vi "Controller LNLS Control PS Communication Loop.vi"(7 "Sync Objects":T1, 8 "error in (no error)":errorcluster, 11 "FOFB Configuration":T5={"FOFB Parameters"={"Network"={"FOFB Controller IP"="", "LNLS Control Network IP"="", "LNLS Control Network Power Supplies TCP Port"=0, "LNLS Control Network FOFB Configuration TCP Port"=0, "Data Server TCP Port"=0, "Monitoring Data TCP Port"=0, "Configuration GUI TCP Port"=0, "TCP Listening Timeout"=0}, "Fast Acquisition"={"Acquisition Period"=0, "Data Buffer Size"=0}, "Response Matrix Measurement"={"Step Amplitude"=0.0, "Time Between Steps"=0, "Step Duration"=0, "Number of Averages"=0}, "Correction Algorithm"={"Correction Period"=0, "Reference Orbit Path"=path "", "Response Matrix Path"=path "", "Correction Matrix Path"=path "", "Horizontal Correction Factor"=0.0, "Vertical Correction Factor"=0.0, "Beam Current FOFB Threshold"=0.0, "Decouple H-V"=FALSE}, "Acquisition Network"=[], "Actuation Network"=[]}, "Number of Acquisition Chassis"=0, "Number of Actuation Chassis"=0, "Number of BPM Readings"=0, "BPM Reading Names"=[], "Selected BPM Readings"=[0, 1, 2, 3, 4, 5, 6, 7, 8, 9, 10, 11, 12, 13, 14, 15, 16, 17, 18, 19, 20, 21, 22, 23, 24, 25, 26, 27, 28, 29, 30, 31, 32, 33, 34, 35, 36, 37, 38, 39, 40, 41, 42, 43, 44, 45, 46, 47, 48, 49], "Number of Correctors"=0, "Corrector Names"=[], "Selected Correctors"=[0, 1, 2, 3, 4, 5, 6, 7, 8, 9, 10, 11, 12, 13, 14, 15, 16, 17, 18, 19, 20, 21, 22, 23, 24, 25, 26, 27, 28, 29, 30, 31, 32, 33, 34, 35, 36, 37, 38, 39, 40, 41, 42, 43, 44, 45, 46, 47, 48, 49], "Reference Orbit"=[], "Response Matrix"=[], "Correction Matrix"=[], "Acquisition Chassis Names"=[], "Actuation Chassis Names"=[], "Acquisition Variables"=[], "Actuation Variables"=[], "PS Matrix Mapping"=[], "Inverse PS Matrix Mapping"=[], "Response Matrix Beam Energy (MeV)"=0.0, "PID Parameters"=[], "BPM Planes"=[], "Corrector Planes"=[], "RMM Step Factor"=[]}) -> (0 "error out":errorcluster)   [LabVIEW 2011, in "Controller VIs.lvlib"]
uses:
  Controller VIs.lvlib
  Types Definitions/Type FOFB Configuration.ctl
  Types Definitions/Type FOFB Parameters.ctl
  Types Definitions/Type Network Configuration.ctl
  Types Definitions/Type FA Configuration.ctl
  Types Definitions/Type Response Matrix Measurement Configuration.ctl
  Types Definitions/Type Correction Algorithm Configuration.ctl
  Types Definitions/Type Acquisition Network Configuration.ctl
  Types Definitions/Type Actuation Network Configuration.ctl
  Types Definitions/Type PID Parameters.ctl
  Types Definitions/Type Synchronization Objects.ctl
  Types Definitions/Type Blocking Synchronization Objects.ctl
  Types Definitions/Type FA Request Parameters.ctl
  Types Definitions/Type BPM and PS select cluster.ctl
  Types Definitions/Type FA File Parameters.ctl
  Types Definitions/Type Monitoring Data.ctl
  Types Definitions/Type Diagnostics Data.ctl
  Types Definitions/Type CPU Loads Array.ctl
  Types Definitions/Type CPU Loads.ctl
  Types Definitions/Type Non-blocking Synchronization Objects.ctl
  Types Definitions/Type FOFB Variables.ctl
  Types Definitions/Type Actuation State.ctl
  <vilib>/Platform/TimedLoop/XDataNode/timing_clust.ctl
  <vilib>/Platform/TimedLoop/XDataNode/nitl_modes.ctl
  <vilib>/Platform/TimedLoop/XDataNode/wakeup.ctl
  Controller Global Variables/Monitoring Data.vi
  <vilib>/Platform/TimedLoop/XDataNode/XDataNode.xnode
  LNLS Control VIs.lvlib
  Common VIs.lvlib
  Misc VIs.lvlib
  Controller Global Variables.lvlib
  <vilib>/Platform/TimedLoop/XDataNode/XDNodeRunTimeDep.lvlib
  Log VIs.lvlib
  Type Definitions.lvlib
panel:
  out "Comando 1":u8[](array[numeric])
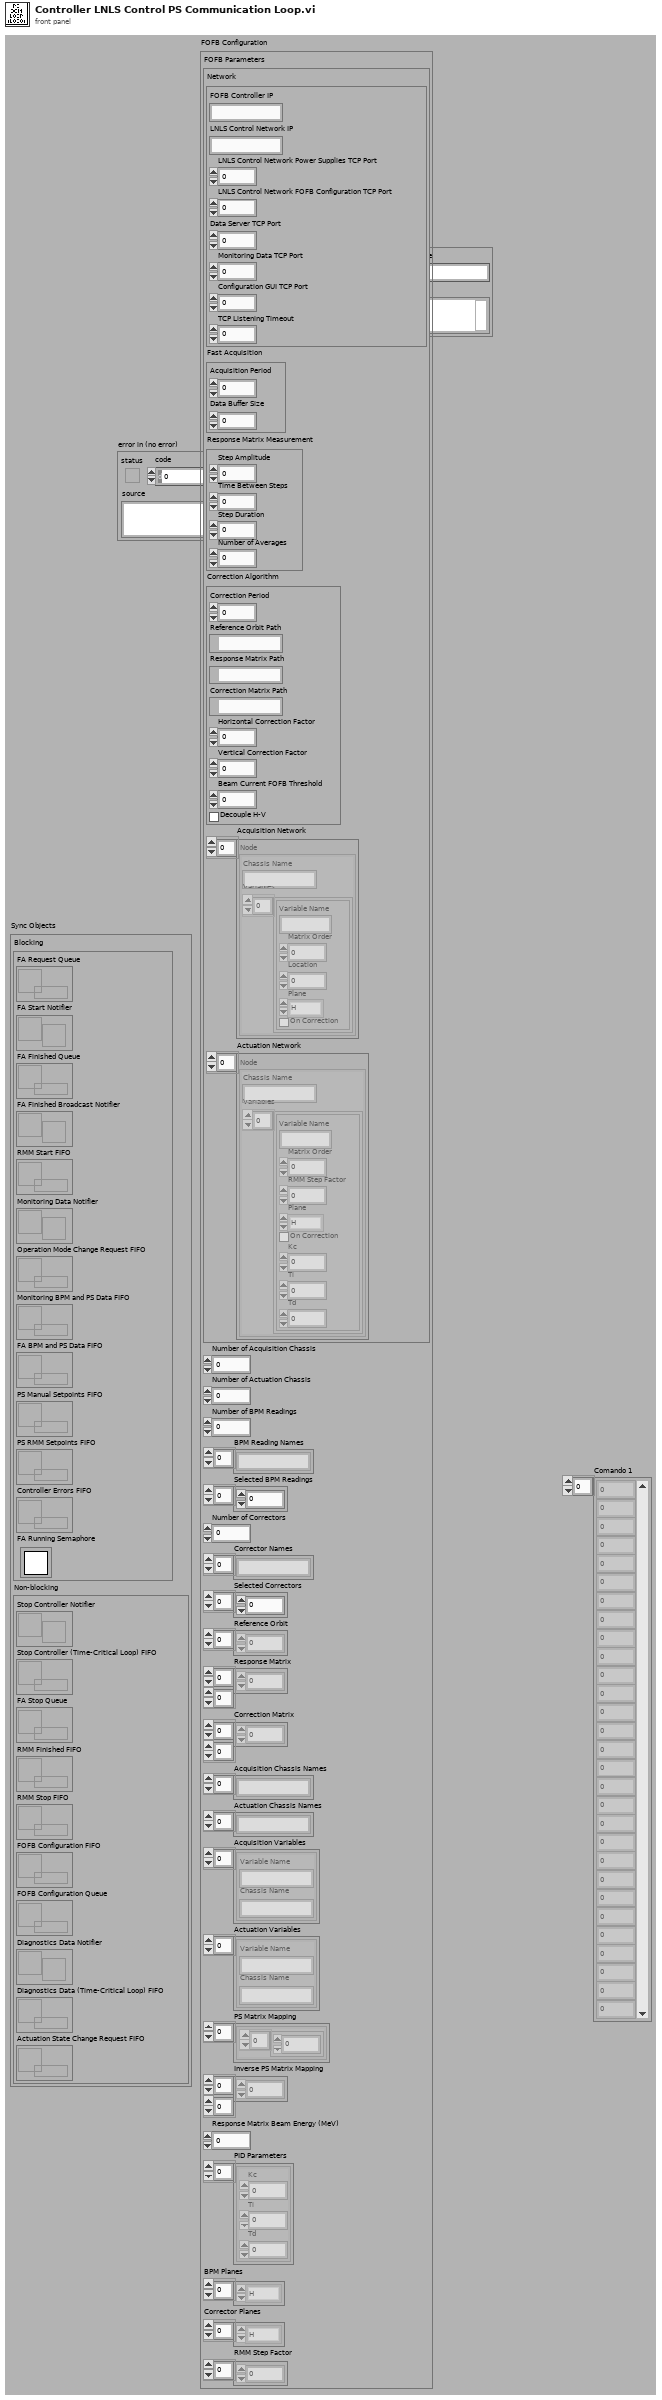
[diagram p1: front panel]
types:
  T1 = typedef "Type Definitions.lvlib/Type Synchronization Objects.ctl" = cluster{"Blocking":T2, "Non-blocking":T4}
  T2 = typedef "Type Definitions.lvlib/Type Blocking Synchronization Objects.ctl" = cluster{"FA Request Queue":refnum<queue>, "FA Start Notifier":refnum<notifier>, "FA Finished Queue":refnum<queue>, "FA Finished Broadcast Notifier":refnum<notifier>, "RMM Start FIFO":refnum<k33>, "Monitoring Data Notifier":refnum<notifier>, "Operation Mode Change Request FIFO":refnum<k33>, "Monitoring BPM and PS Data FIFO":refnum<k33>, "FA BPM and PS Data FIFO":refnum<k33>, "PS Manual Setpoints FIFO":refnum<k33>, "PS RMM Setpoints FIFO":refnum<k33>, "Controller Errors FIFO":refnum<k33>, "FA Running Semaphore":T3}
  T3 = typedef "Semaphore RefNum" = refnum<k1>
  T4 = typedef "Type Definitions.lvlib/Type Non-blocking Synchronization Objects.ctl" = cluster{"Stop Controller Notifier":refnum<notifier>, "Stop Controller (Time-Critical Loop) FIFO":refnum<k33>, "FA Stop Queue":refnum<queue>, "RMM Finished FIFO":refnum<k33>, "RMM Stop FIFO":refnum<k33>, "FOFB Configuration FIFO":refnum<k33>, "FOFB Configuration Queue":refnum<queue>, "Diagnostics Data Notifier":refnum<notifier>, "Diagnostics Data (Time-Critical Loop) FIFO":refnum<k33>, "Actuation State Change Request FIFO":refnum<k33>}
  T5 = typedef "Type Definitions.lvlib/Type FOFB Configuration.ctl" = cluster{"FOFB Parameters":T6, "Number of Acquisition Chassis":i32, "Number of Actuation Chassis":i32, "Number of BPM Readings":i32, "BPM Reading Names":string[], "Selected BPM Readings":u32[], "Number of Correctors":i32, "Corrector Names":string[], "Selected Correctors":u32[], "Reference Orbit":dbl[], "Response Matrix":dbl[][], "Correction Matrix":dbl[][], "Acquisition Chassis Names":string[], "Actuation Chassis Names":string[], "Acquisition Variables":cluster{"Variable Name":string, "Chassis Name":string}[], "Actuation Variables":cluster{"Variable Name":string, "Chassis Name":string}[], "PS Matrix Mapping":cluster{u32[]}[], "Inverse PS Matrix Mapping":u32[][], "Response Matrix Beam Energy (MeV)":dbl, "PID Parameters":T13[], "BPM Planes":enum8{"H", "V"}[], "Corrector Planes":enum8{"H", "V"}[], "RMM Step Factor":dbl[]}
  T6 = typedef "Type Definitions.lvlib/Type FOFB Parameters.ctl" = cluster{"Network":T7, "Fast Acquisition":T8, "Response Matrix Measurement":T9, "Correction Algorithm":T10, "Acquisition Network":T11, "Actuation Network":T12}
  T7 = typedef "Type Definitions.lvlib/Type Network Configuration.ctl" = cluster{"FOFB Controller IP":string, "LNLS Control Network IP":string, "LNLS Control Network Power Supplies TCP Port":u16, "LNLS Control Network FOFB Configuration TCP Port":u16, "Data Server TCP Port":u16, "Monitoring Data TCP Port":u16, "Configuration GUI TCP Port":u16, "TCP Listening Timeout":i32}
  T8 = typedef "Type Definitions.lvlib/Type FA Configuration.ctl" = cluster{"Acquisition Period":u32, "Data Buffer Size":u32}
  T9 = typedef "Type Definitions.lvlib/Type Response Matrix Measurement Configuration.ctl" = cluster{"Step Amplitude":dbl, "Time Between Steps":u32, "Step Duration":u32, "Number of Averages":u32}
  T10 = typedef "Type Definitions.lvlib/Type Correction Algorithm Configuration.ctl" = cluster{"Correction Period":u32, "Reference Orbit Path":path, "Response Matrix Path":path, "Correction Matrix Path":path, "Horizontal Correction Factor":dbl, "Vertical Correction Factor":dbl, "Beam Current FOFB Threshold":dbl, "Decouple H-V":bool}
  T11 = typedef "Type Definitions.lvlib/Type Acquisition Network Configuration.ctl" = cluster{"Chassis Name":string, "Variables":cluster{"Variable Name":string, "Matrix Order":u32, "Location":dbl, "Plane":enum8{"H", "V"}, "On Correction":bool}[]}[]
  T12 = typedef "Type Definitions.lvlib/Type Actuation Network Configuration.ctl" = cluster{"Chassis Name":string, "Variables":cluster{"Variable Name":string, "Matrix Order":u32, "RMM Step Factor":dbl, "Plane":enum8{"H", "V"}, "On Correction":bool, "Kc":dbl, "Ti":dbl, "Td":dbl}[]}[]
  T13 = typedef "Type Definitions.lvlib/Type PID Parameters.ctl" = cluster{"Kc":fxp<+/-,16,8>, "Ti":fxp<+/-,16,8>, "Td":fxp<+/-,16,8>}
  T14 = enum16{"Wait Connection", "Read Data", "Write Data", "Close Connection", "Idle"}
  T15 = typedef "XDNodeRunTimeDep.lvlib/timing_clust.ctl" = cluster{"Expected End [f-1]":u64, "Actual End [f-1]":u64, "Finished Late? [f-1]":bool, "Expected End [i-1]":u64, "Actual End [i-1]":u64, "Finished Late? [i-1]":bool, "Expected Start [i]":u64, "Actual Start [i]":u64, "Expected Start [f]":u64, "Actual Start [f]":u64, "Source Name":string, "Structure Name":string, "Period":i64, "Deadline":i64, "Offset":i64, "Start":i64, "Priority":i32, "Timeout":i32, "Mode":T16, "Wakeup Reason":T17, "Error":errorcluster, "Source Type":string, "Secondary Source Type":string, "Global End Time":u64, "Global Start Time":u64, "Frame Duration":u64, "Iteration Duration":u64, "Assigned CPU":i32, "I/O Scan Engine Mode":u32}
  T16 = typedef "XDNodeRunTimeDep.lvlib/nitl_modes.ctl" = enum32{"No Change", "Process missed periods, maintain original phase", "Discard missed periods, maintain original phase", "Process missed periods, ignore original phase", "Discard missed periods, ignore original phase"}
  T17 = typedef "XDNodeRunTimeDep.lvlib/wakeup.ctl" = enum32{"Normal", "Aborted", "Asynchronous wakeup", "Timing source error", "Timed loop error", "Timeout"}
  T18 = enum16{"open", "replace", "create", "open or create", "replace or create", "replace or create with confirmation"}
  T19 = typedef "Type Definitions.lvlib/Type Monitoring Data.ctl" = cluster{"Timestamp":timestamp, "BPM Readings":dbl[], "PS Readings":dbl[], "PS FOFB Setpoints":dbl[], "PS Status per Rack":u8[], "PS ON-OFF per Rack":u8[], "Operation Mode":enum16{"Idle Mode", "Error Mode", "Manual Mode", "FOFB Mode", "RMM Mode"}, "Diagnostics Data":T20, "Controller Status Table":i32[]}
  T20 = typedef "Type Definitions.lvlib/Type Diagnostics Data.ctl" = cluster{"Time-Critical Loop Missed Iterations":u32, "Time-Critical Loop Execution Time (usec)":u32, "FA Buffer Usage":u32, "Available Memory (bytes)":u32, "CPU Loads Array":T21}
  T21 = typedef "Type Definitions.lvlib/Type CPU Loads Array.ctl" = T22[]
  T22 = typedef "Type Definitions.lvlib/Type CPU Loads.ctl" = cluster{"Total (%)":dbl, "Time Critical (%)":dbl, "Timed Structures (%)":dbl, "High (%)":dbl, "Above Normal (%)":dbl, "Normal (%)":dbl, "Background (%)":dbl, "Idle (%)":dbl, "ISR (%)":dbl}
  T23 = typedef "Type Definitions.lvlib/Type LOCON_BIPOLAR_16BITS.ctl" = cluster{"priority":u8, "flag":u8, "analog value":u16, "status":u8}
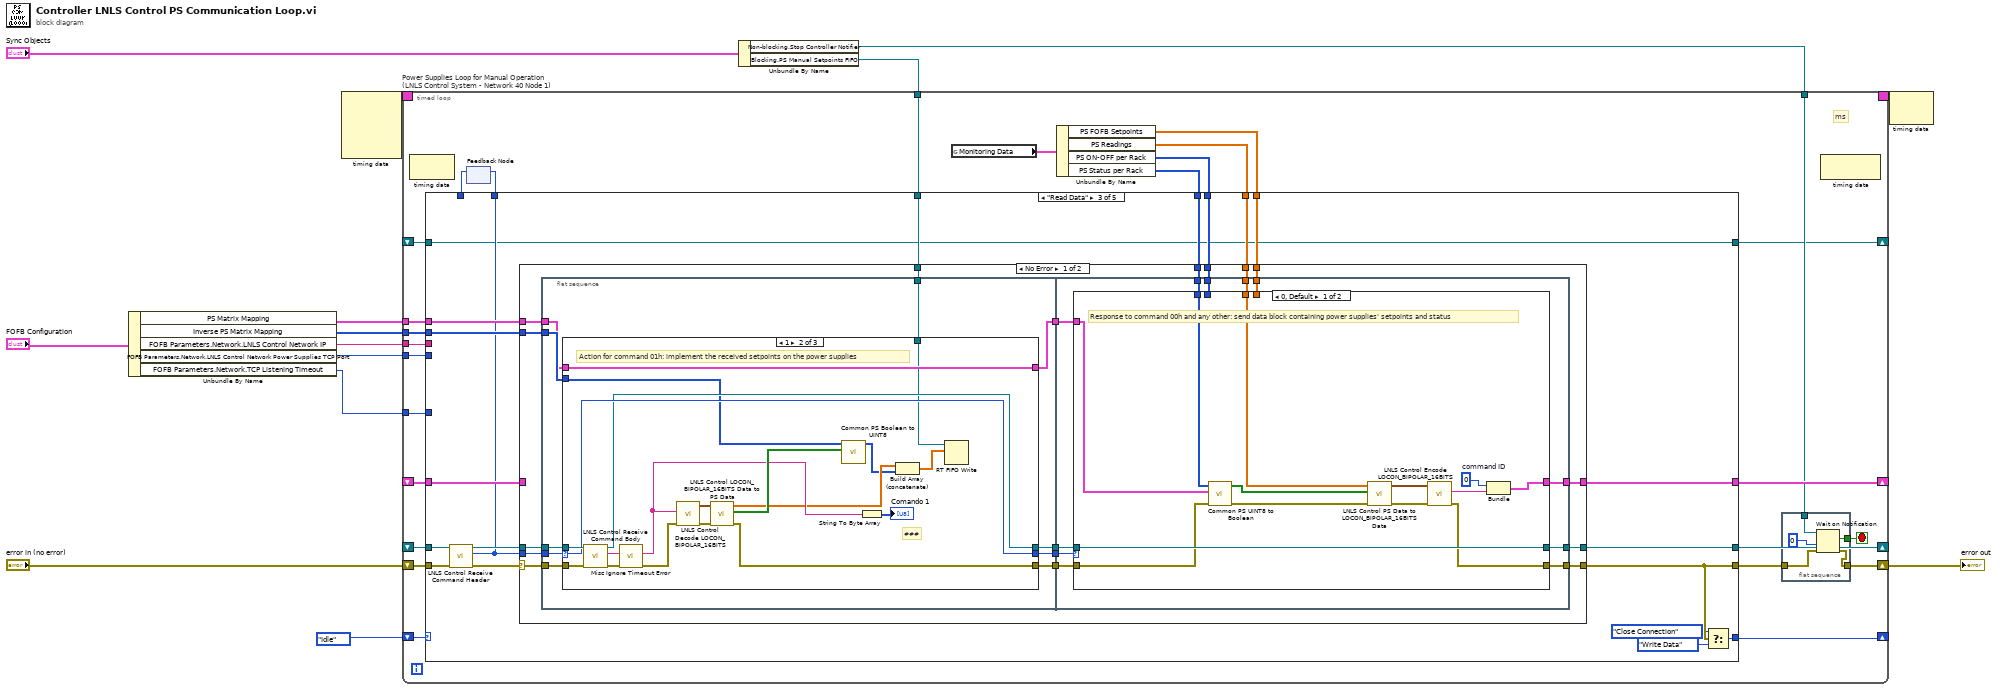
[diagram p0: block diagram]
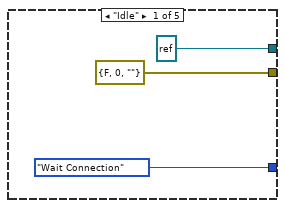
[diagram p2: hidden frame]
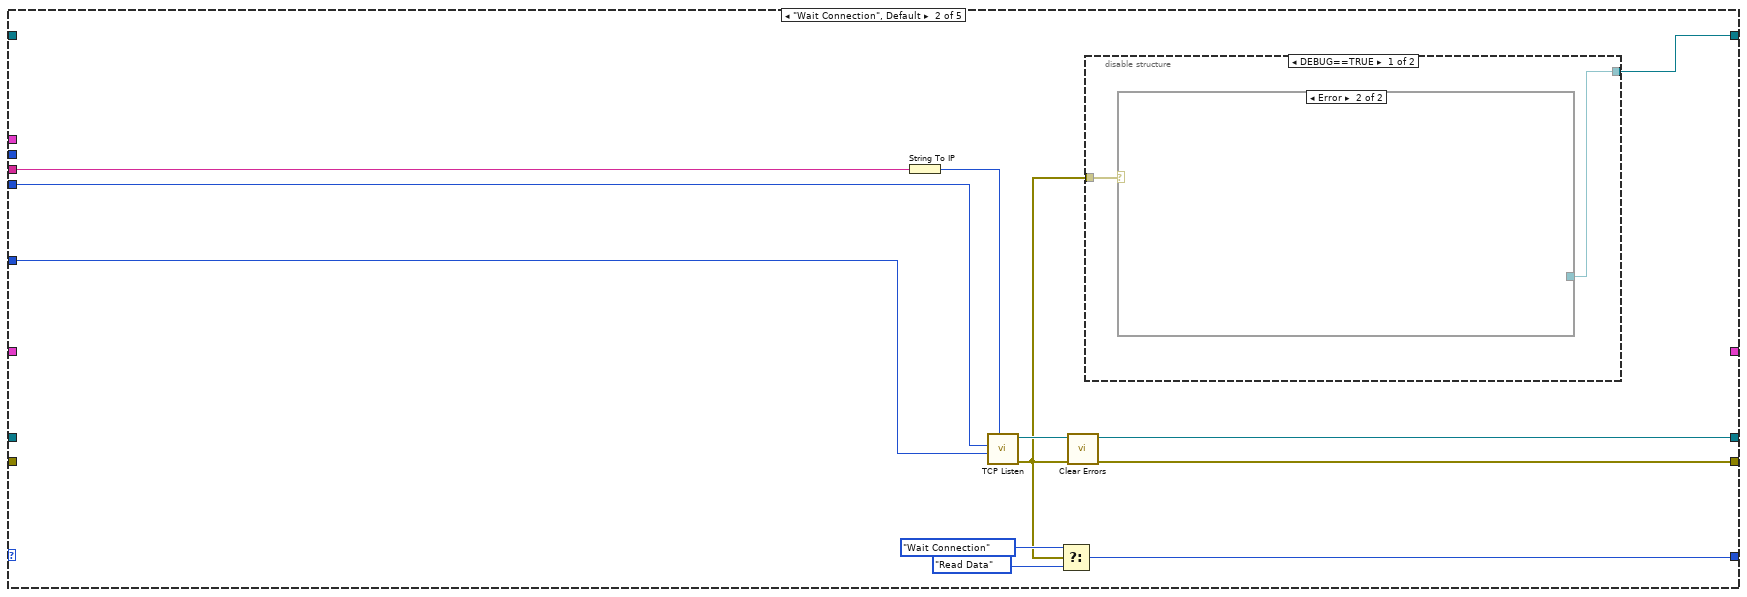
[diagram p3: hidden frame]
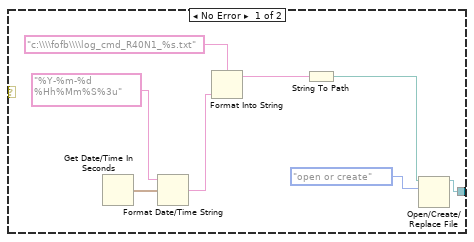
[diagram p4: hidden frame]
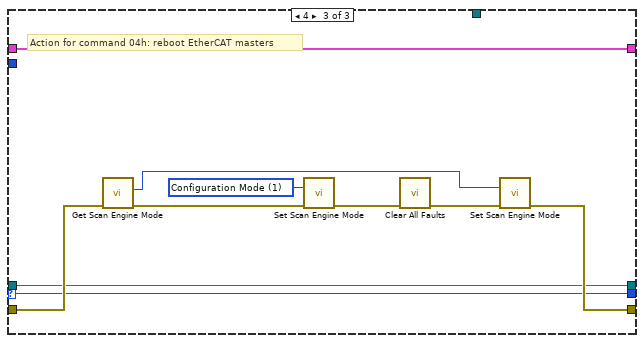
[diagram p7: hidden frame]
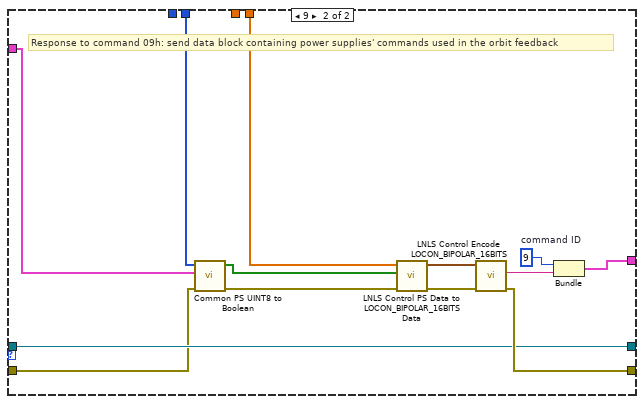
[diagram p8: hidden frame]
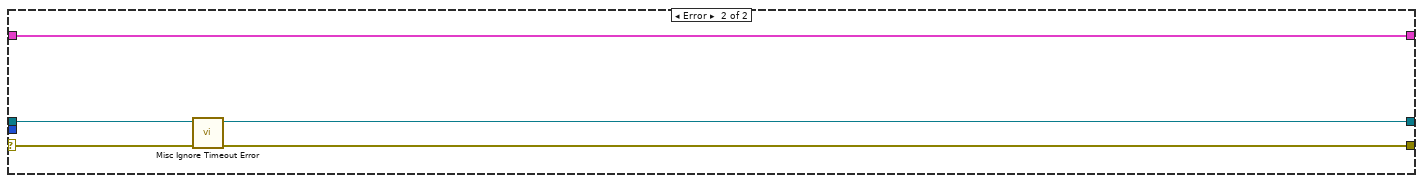
[diagram p9: hidden frame]
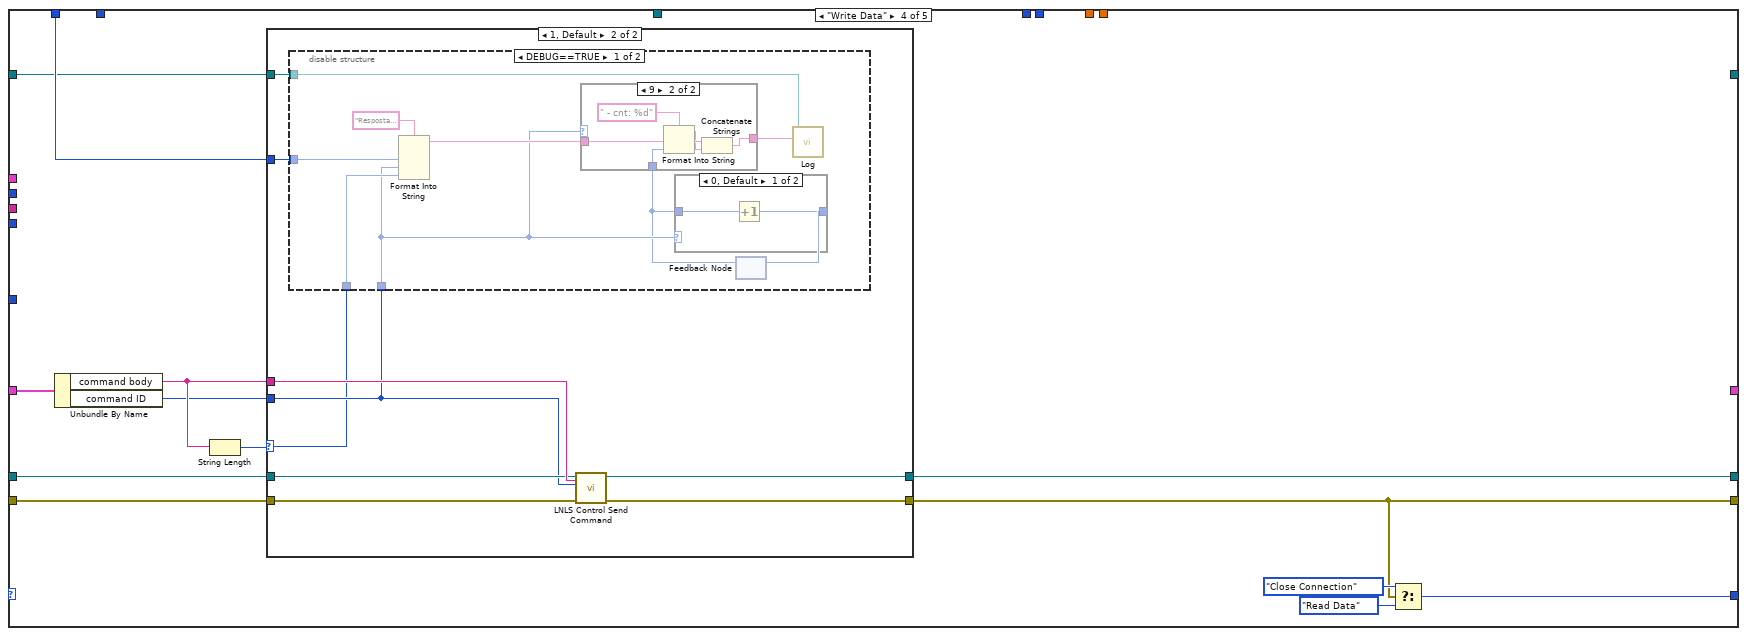
[diagram p10: hidden frame]
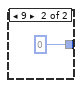
[diagram p13: hidden frame]
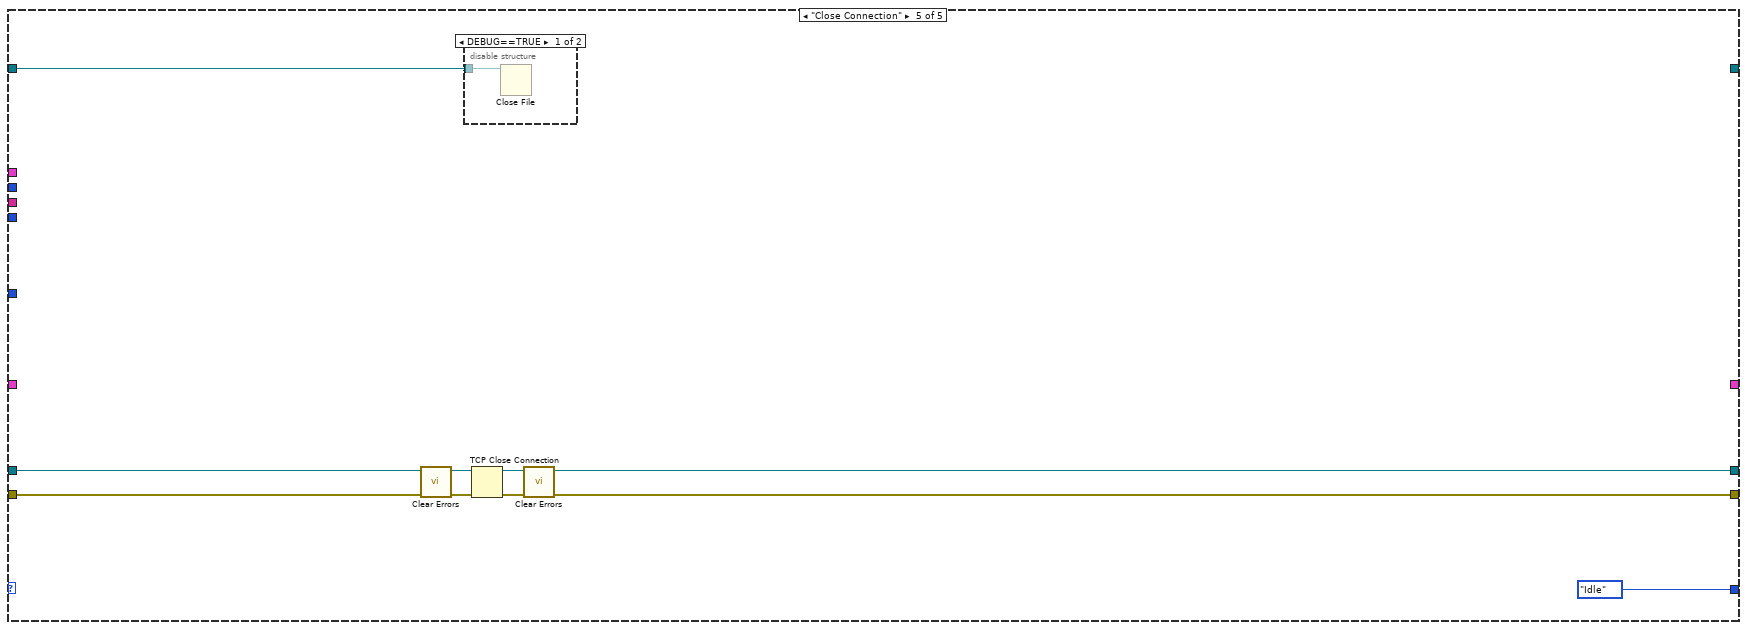
[diagram p15: hidden frame]
diagram:
  n1 = Unbundle By Name("FOFB Configuration") -> ("PS Matrix Mapping"=w7:cluster{u32[]}[], "Inverse PS Matrix Mapping"=w8:u32[][], "FOFB Parameters.Network.LNLS Control Network IP"=w9:string, "FOFB Parameters.Network.LNLS Control Network Power Supplies TCP Port"=w6:u16, "FOFB Parameters.Network.TCP Listening Timeout"=w4:i32)
  n2 = node-c288() -> (w2:T15)  [unwired: 4 in]
  n3 = Unbundle By Name("Sync Objects") -> ("Non-blocking.Stop Controller Notifier"=w5:refnum<notifier>, "Blocking.PS Manual Setpoints FIFO"=w3:refnum<k33>)
  n4 = timed-loop "Power Supplies Loop for Manual Operation (LNLS Control System - Network 40 Node 1)" {
    shift-right: [w38] -> _
    shift-left: T14."Idle" ("f") -> [w40]
    shift-right: [w39] -> _
    shift-left: _ -> [w37]
    shift-right: [w25] -> w12
    shift-left: "error in (no error)" -> [w33]
    shift-right: [w35] -> _
    shift-left: _ -> [w34]
    tunnel: w6 -> [w36]
    tunnel: w9 -> [w32]
    tunnel: w8 -> [w31]
    tunnel: w7 -> [w30]
    tunnel: w5 -> [w28]
    tunnel: w4 -> [w29]
    tunnel: w3 -> [w21]
    timing: w2 -> [_]
    timing-out: [_] -> w1
    shift-right: [w16] -> _
    shift-left: _ -> [w15]
    stop <- w27 stop-if-true
    # "ms"
    n5 = node-c288() -> ()  [unwired: 1 in, 1 out]
    n6 = feedback #1() -> (w17:u8)  [unwired: 1 in]
    n7 = global read "Monitoring Data.vi" "Monitoring Data"() -> (w22:T19)
    n8 = Unbundle By Name(w22) -> ("PS FOFB Setpoints"=w24:dbl[], "PS Readings"=w23:dbl[], "PS ON-OFF per Rack"=w19:u8[], "PS Status per Rack"=w20:u8[])
    n9 = case shown="\"Read Data\"" w40 {
      tunnel: [refnum<k5> refnum ("connection ID") w57 w91 w197 w240] -> w39
      tunnel: [errorcluster {"status"=FALSE, "code"=0, "source"=""} ("error out") w60 w89 w196 w237] -> w26
      tunnel: [T14."Wait Connection" w61 w90 w202 T14."Idle"] -> w38
      tunnel: w37 -> [_ _ w87 w199 w241]
      tunnel: w33 -> [_ _ w88 w198 w235]
      tunnel: w36 -> [_ w56 _ _ _]
      tunnel: [_ _ w84 _ _] -> w35
      tunnel: w34 -> [_ _ w82 w201 _]
      tunnel: w32 -> [_ w54 _ _ _]
      tunnel: w31 -> [_ _ w80 _ _]
      tunnel: w30 -> [_ _ w79 _ _]
      tunnel: w29 -> [_ w53 _ _ _]
      tunnel: w24 -> [_ _ w78 _ _]
      tunnel: w23 -> [_ _ w77 _ _]
      tunnel: w20 -> [_ _ w76 _ _]
      tunnel: w21 -> [_ _ w75 _ _]
      tunnel: w19 -> [_ _ w74 _ _]
      tunnel: w17 -> [_ _ _ w194 _]
      tunnel: [_ _ w73 _ _] -> w18
      tunnel: [_ w52 w72 _ _] -> w16
      tunnel: w15 -> [_ _ w72 w193 w234]
      frame "Idle" {
      }
      frame "Wait Connection", Default {
        n10 = String To IP(1:w54) -> (0:w55:u32)
        n11 = call <vilib>:"TCP Listen.vi"("net address"=w55, "timeout ms (wait forever: -1)"=w53, "port"=w56) -> ("error out"=w51:errorcluster, "connection ID"=w57:refnum<k5>)  [unwired: 4 in, 3 out]
        n12 = Select(t=T14."Wait Connection", s=w51, f=T14."Read Data") -> (s? t:f=w61:T14)
        n13 = call <vilib>:"Clear Errors.vi"("error in (no error)"=w51) -> ("error out"=w60:errorcluster)  [unwired: 6 out]
        n14 = disable-structure shown="DEBUG==TRUE" {
          disable-tunnel: [w63 _] -> w52
          disable-tunnel: w51 -> [w62 _]
          frame condition #0 {
            n15 = case shown="Error" w62 {
              tunnel: [w64 _] -> w63
              frame No Error {
                n16 = Get Date/Time In Seconds() -> (seconds since 1Jan1904=w67:timestamp)
                n17 = Format Date/Time String(time format string (%c)="%Y-%m-%d %Hh%Mm%S%3u", seconds (now)=w67) -> (date/time string=w65:string)  [unwired: 1 in]
                n18 = Format Into String(format string="c:\\\\fofb\\\\log_cmd_R40N1_%s.txt", w65) -> (resulting string=w69:string)  [unwired: 2 in, 1 out]
                n19 = String To Path(string=w69) -> (path=w68:path)
                n20 = Open/Create/Replace File(file path (use dialog)=w68, operation (0:open)=T18."open or create") -> (refnum out=w64:refnum<file>)  [unwired: 4 in, 2 out]
              }
              frame Error {
              }
            }
          }
          frame condition #1 (active) {
          }
        }
      }
      frame "Read Data" {
        n21 = call "LNLS Control Receive Command Header.vi"("error in (no error)"=w88, "connection ID"=w87) -> ("error out"=w83:errorcluster, "command ID"=w73:u8, "connection ID out"=w86:refnum<k5>)  [unwired: 7 in]
        n22 = case shown="No Error" w83 {
          selector: w83 -> [w103 w188]
          tunnel: [w108 w191] -> w91
          tunnel: [w107 w189] -> w89
          tunnel: w86 -> [w106 w191]
          tunnel: w73 -> [w105 _]
          tunnel: [w104 w190] -> w84
          tunnel: w82 -> [_ w190]
          tunnel: w80 -> [w99 _]
          tunnel: w79 -> [w97 _]
          tunnel: w78 -> [w96 _]
          tunnel: w77 -> [w95 _]
          tunnel: w76 -> [w94 _]
          tunnel: w75 -> [w93 _]
          tunnel: w74 -> [w92 _]
          frame No Error {
            n23 = flat-sequence {
              tunnel: [w118] -> w102
              tunnel: [w117] -> w101
              tunnel: w106 -> [w116]
              tunnel: w105 -> [w115]
              tunnel: w103 -> [w114]
              tunnel: [w113] -> w100
              tunnel: w99 -> [w112]
              tunnel: [w111] -> w98
              tunnel: w97 -> [w110]
              tunnel: w93 -> [w109]
              tunnel: [w158] -> w108
              tunnel: w102 -> [w157]
              tunnel: [w161] -> w107
              tunnel: w101 -> [w160]
              tunnel: [w156] -> w104
              tunnel: w100 -> [w159]
              tunnel: w98 -> [w155]
              tunnel: w96 -> [w154]
              tunnel: w95 -> [w153]
              tunnel: w94 -> [w152]
              tunnel: w92 -> [w151]
              frame #0 {
                n24 = case shown="1" w115 {
                  selector: w115 -> [w120 w137 w143]
                  tunnel: w114 -> [w122 w139 w150]
                  tunnel: [w122 w138 w149] -> w117
                  tunnel: [w121 w136 w142] -> w118
                  tunnel: w116 -> [w121 w140 w142]
                  tunnel: [w120 w137 w143] -> w113
                  tunnel: w112 -> [_ w135 _]
                  tunnel: [w119 w134 w141] -> w111
                  tunnel: w110 -> [w119 w134 w141]
                  tunnel: w109 -> [_ w126 _]
                  frame 0, Default {
                  }
                  frame 1 {
                    # "###"
                    # "Action for command 01h: implement the received setpoints on the power supplies"
                    n25 = call "LNLS Control Receive Command Body.vi"("error in (no error)"=w139, "connection ID"=w140) -> ("error out"=w130:errorcluster, "command body"=w128:string, "connection ID out"=w136:refnum<k5>)  [unwired: 6 in, 1 out]
                    n26 = call "Misc Ignore Timeout Error.vi"("error in (no error)"=w130) -> ("error out"=w129:errorcluster)  [unwired: 10 in]
                    n27 = call "LNLS Control Decode LOCON_BIPOLAR_16BITS.vi"("error in (no error)"=w129, "command body"=w128) -> ("error out"=w133:errorcluster, "LOCON data"=w132:T23[])  [unwired: 6 in]
                    n28 = call "LNLS Control LOCON_BIPOLAR_16BITS Data to PS Data.vi"("error in (no error)"=w133, "PS Setpoints LOCON Data"=w132) -> ("error out"=w138:errorcluster, "PS Status"=w131:bool[], "PS Setpoints"=w125:dbl[])  [unwired: 7 in]
                    n29 = call "Common PS Boolean to UINT8.vi"("PS ON-OFF"=w131, "Inverse PS Matrix Mapping"=w135) -> ("PS ON-OFF (per PS Rack)"=w124:u8[])  [unwired: 8 in, 1 out]
                    n30 = String To Byte Array(string=w128) -> (unsigned byte array=→"Comando 1":u8[])
                    n31 = Build Array (concatenate)(w125, w124) -> (w123:dbl[])
                    n32 = RT FIFO Write(0:w126, 1:w123) -> ()  [unwired: 3 in, 4 out]
                  }
                  frame 4 {
                    w148 = 1 items=["Configuration Mode"=1, "Active Mode"=2] ("mode (Active Mode)")
                    # "Action for command 04h: reboot EtherCAT masters"
                    n33 = call <vilib>:"Get Scan Engine Mode.vi"("error in (no error)"=w150) -> ("error out"=w147:errorcluster, "mode"=w144:i32)  [unwired: 9 in]
                    n34 = call <vilib>:"Set Scan Engine Mode.vi"("mode (Active Mode)"=w148, "error in (no error)"=w147) -> ("error out"=w146:errorcluster)  [unwired: 13 in]
                    n35 = call <vilib>:"Clear All Faults.vi"("error in (no error)"=w146) -> ("error out"=w145:errorcluster)  [unwired: 1 in, 9 out]
                    n36 = call <vilib>:"Set Scan Engine Mode.vi"("mode (Active Mode)"=w144, "error in (no error)"=w145) -> ("error out"=w149:errorcluster)  [unwired: 13 in]
                  }
                }
              }
              frame #1 {
                n37 = case shown="0, Default" w159 {
                  tunnel: w160 -> [w168 w182]
                  tunnel: [w169 w185] -> w161
                  tunnel: [w174 w184] -> w158
                  tunnel: w157 -> [w174 w184]
                  tunnel: [w170 w183] -> w156
                  tunnel: w155 -> [w166 w180]
                  tunnel: w154 -> [_ w178]
                  tunnel: w153 -> [w163 _]
                  tunnel: w152 -> [w162 _]
                  tunnel: w151 -> [_ w175]
                  frame 0, Default {
                    w171 = u8 0  # command ID
                    # "Response to command 00h and any other: send data block containing power supplies' setpoints and status"
                    n38 = call "Common PS UINT8 to Boolean.vi"("error in (no error)"=w168, "PS Matrix Mapping"=w166, "PS Status (per PS Rack)"=w162) -> ("error out"=w165:errorcluster, "PS Status"=w167:bool[])  [unwired: 7 in]
                    n39 = call "LNLS Control PS Data to LOCON_BIPOLAR_16BITS Data.vi"("error in (no error)"=w165, "PS Status"=w167, "PS Readings/Setpoints"=w163) -> ("error out"=w172:errorcluster, "PS Readings/Setpoints LOCON Data"=w173:T23[])  [unwired: 7 in]
                    n40 = call "LNLS Control Encode LOCON_BIPOLAR_16BITS.vi"("error in (no error)"=w172, "LOCON Data"=w173) -> ("error out"=w169:errorcluster, "command body"=w164:string)  [unwired: 8 in]
                    n41 = Bundle("command ID"=w171, "command body"=w164) -> (w170:cluster{"command ID":u8, "command body":string})  [unwired: 1 in]
                  }
                  frame 9 {
                    w186 = u8 9  # command ID
                    # "Response to command 09h: send data block containing power supplies' commands used in the orbit feedback"
                    n42 = call "Common PS UINT8 to Boolean.vi"("error in (no error)"=w182, "PS Matrix Mapping"=w180, "PS Status (per PS Rack)"=w175) -> ("error out"=w179:errorcluster, "PS Status"=w181:bool[])  [unwired: 7 in]
                    n43 = call "LNLS Control PS Data to LOCON_BIPOLAR_16BITS Data.vi"("error in (no error)"=w179, "PS Status"=w181, "PS Readings/Setpoints"=w178) -> ("error out"=w176:errorcluster, "PS Readings/Setpoints LOCON Data"=w177:T23[])  [unwired: 7 in]
                    n44 = call "LNLS Control Encode LOCON_BIPOLAR_16BITS.vi"("error in (no error)"=w176, "LOCON Data"=w177) -> ("error out"=w185:errorcluster, "command body"=w187:string)  [unwired: 8 in]
                    n45 = Bundle("command ID"=w186, "command body"=w187) -> (w183:cluster{"command ID":u8, "command body":string})  [unwired: 1 in]
                  }
                }
              }
            }
          }
          frame Error {
            n46 = call "Misc Ignore Timeout Error.vi"("error in (no error)"=w188) -> ("error out"=w189:errorcluster)  [unwired: 10 in]
          }
        }
        n47 = Select(t=T14."Close Connection", s=w89, f=T14."Write Data") -> (s? t:f=w90:T14)
      }
      frame "Write Data" {
        n48 = Unbundle By Name(w201) -> ("command body"=w200:string, "command ID"=w195:u8)
        n49 = String Length(string=w200) -> (length=w192:i32)
        n50 = case shown="1, Default" w192 {
          selector: w192 -> [_ w207]
          tunnel: w200 -> [_ w215]
          tunnel: w199 -> [w206 w214]
          tunnel: w198 -> [w205 w213]
          tunnel: [w206 w212] -> w197
          tunnel: [w205 w211] -> w196
          tunnel: w195 -> [_ w210]
          tunnel: w194 -> [_ w209]
          tunnel: w193 -> [_ w208]
          frame 0 {
          }
          frame 1, Default {
            n51 = disable-structure shown="DEBUG==TRUE" {
              disable-tunnel: w209 -> [w224 _]
              disable-tunnel: w210 -> [w219 _]
              disable-tunnel: w207 -> [w222 _]
              disable-tunnel: w208 -> [w221 _]
              frame condition #0 {
                n52 = Format Into String(format string="Resposta ao cmd #%d - Cmd #%d com %d bytes" ("String"), w224, w219, w222) -> (resulting string=w220:string)  [unwired: 2 in, 1 out]
                n53 = feedback #2() -> (w216:i32)  [unwired: 1 in]
                n54 = case shown="9" w219 {
                  tunnel: w220 -> [w225 w230]
                  tunnel: [w225 w227] -> w218
                  tunnel: w216 -> [_ w226]
                  frame 0, Default {
                  }
                  frame 9 {
                    n55 = Format Into String(format string=" - cnt: %d", w226) -> (resulting string=w229:string)  [unwired: 2 in, 1 out]
                    n56 = Concatenate Strings(w230, w229) -> (w227:string)
                  }
                }
                n57 = case shown="0, Default" w219 {
                  tunnel: [w231 0] -> w217
                  tunnel: w216 -> [w232 _]
                  frame 0, Default {
                    n58 = Increment(x=w232) -> (x+1=w231:i32)
                  }
                  frame 9 {
                  }
                }
                n59 = feedback-in #2(w217) -> ()
                n60 = call "Log.vi"("String"=w218, "Log File Reference"=w221) -> ()  [unwired: 8 in, 2 out]
              }
              frame condition #1 (active) {
              }
            }
            n61 = call "LNLS Control Send Command.vi"("command body"=w215, "error in (no error)"=w213, "command ID"=w210, "connection ID"=w214) -> ("error out"=w211:errorcluster, "connection ID out"=w212:refnum<k5>)  [unwired: 6 in]
          }
        }
        n62 = Select(t=T14."Close Connection", s=w196, f=T14."Read Data") -> (s? t:f=w202:T14)
      }
      frame "Close Connection" {
        n63 = call <vilib>:"Clear Errors.vi"("error in (no error)"=w235) -> ("error out"=w236:errorcluster)  [unwired: 6 in]
        n64 = disable-structure shown="DEBUG==TRUE" {
          disable-tunnel: w234 -> [w242 _]
          frame condition #0 {
            n65 = Close File(refnum=w242) -> ()  [unwired: 1 in, 2 out]
          }
          frame condition #1 (active) {
          }
        }
        n66 = TCP Close Connection(connection ID=w241, error in (no error)=w236) -> (connection ID out=w240:refnum<k5>, error out=w238:errorcluster)  [unwired: 1 in]
        n67 = call <vilib>:"Clear Errors.vi"("error in (no error)"=w238) -> ("error out"=w237:errorcluster)  [unwired: 6 in]
      }
    }
    n68 = feedback-in #1(w18) -> ()
    n69 = flat-sequence {
      tunnel: [w45] -> _
      tunnel: w28 -> [w46]
      tunnel: w26 -> [w44]
      tunnel: [w43] -> w25
      tunnel: [w45] -> w27
      frame #0 {
        n70 = Wait on Notification(notifier=w46, timeout in ms (-1)=0, error in (no error)=w44) -> (notification=w45:bool, error out=w43:errorcluster)  [unwired: 1 in, 2 out]
      }
    }
    n71 = node-c288() -> ()  [unwired: 1 in, 1 out]
  }
  "error out" <- w12
  n72 = node-c288(w1) -> ()  [unwired: 1 out]
